vi "Live Display and capture_4.vi"() -> ()   [LabVIEW 2020]
doc: "The Acquire Every Image (Optimized Performance) example shows the basics of using a ring acquisition. There are some camera restrictions to using this mode that are described in more detail in the block diagram of the VI, but it is recommended to use this method for performance-critical applications when possible."
uses:
  <vilib>/vision/driver/IMAQdx.llb/IMAQdx Acquisition Mode.ctl
  Camera Server/Globals/CamServer global.vi
  <vilib>/vision/driver/NI_Vision_Acquisition_Software.lvlib
  <resource>/objmgr/imaqdx.rc
panel:
  out "Name 4":string
  out "Name 3":string
  out "Name 2":string
  out "Name 1":string
  out "Image 4":T1(plugin-control)
  out "Image 3":T1(plugin-control)
  out "Image 2":T1(plugin-control)
  out "error out":errorcluster
  out "Numeric":i32
  out "Image 1":T1(plugin-control)
  in  "Stop":bool
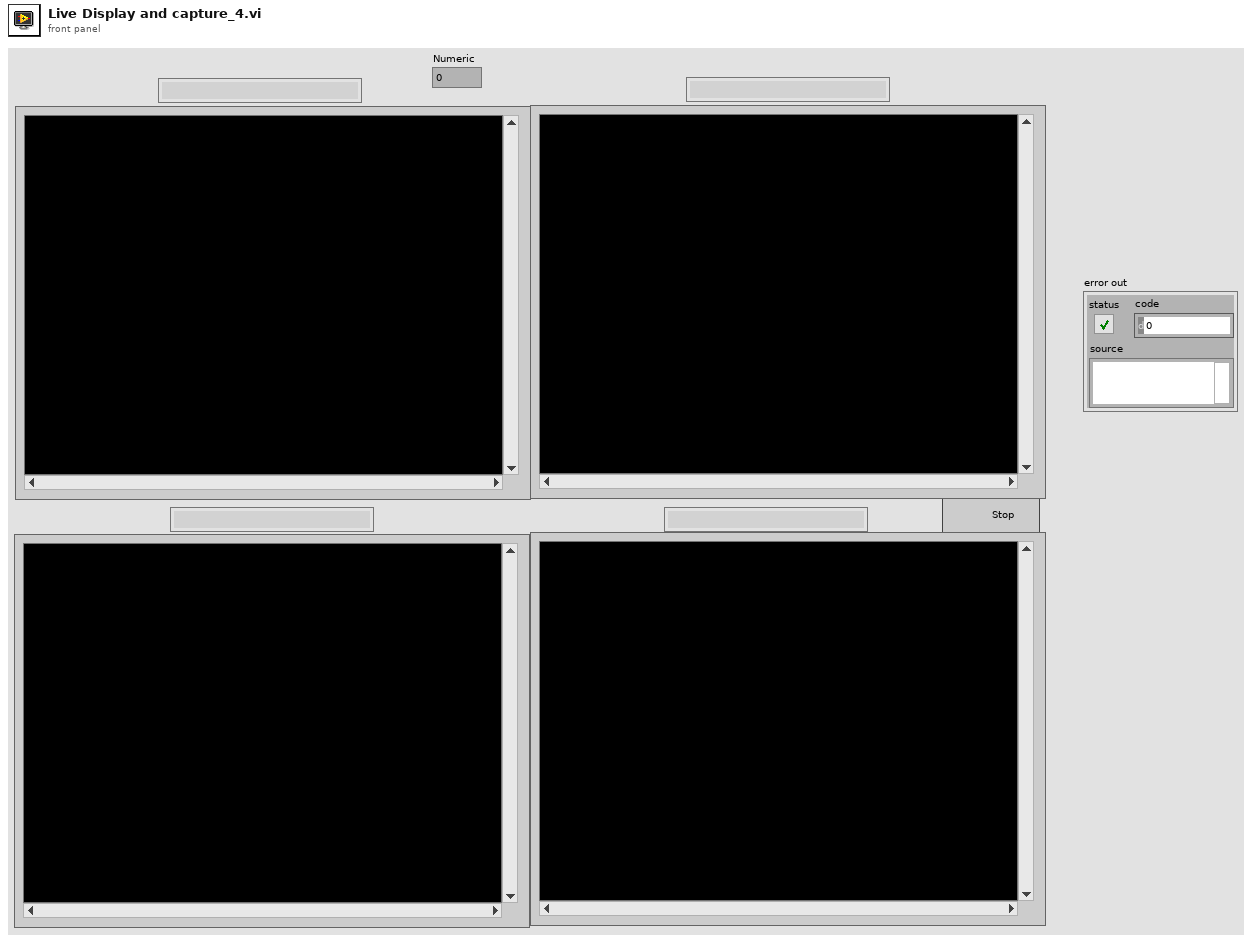
[diagram p1: front panel]
types:
  T1 = typedef "IMAQ Image.ctl" = refnum<image>
  T2 = typedef "NI_Vision_Acquisition_Software.lvlib/IMAQdx Acquisition Mode.ctl" = enum32{"One Shot", "Continuous"}
  T3 = typedef "Camera enum.ctl" = string
  T4 = typedef "IMAQdx.ctl" = refnum<k21>
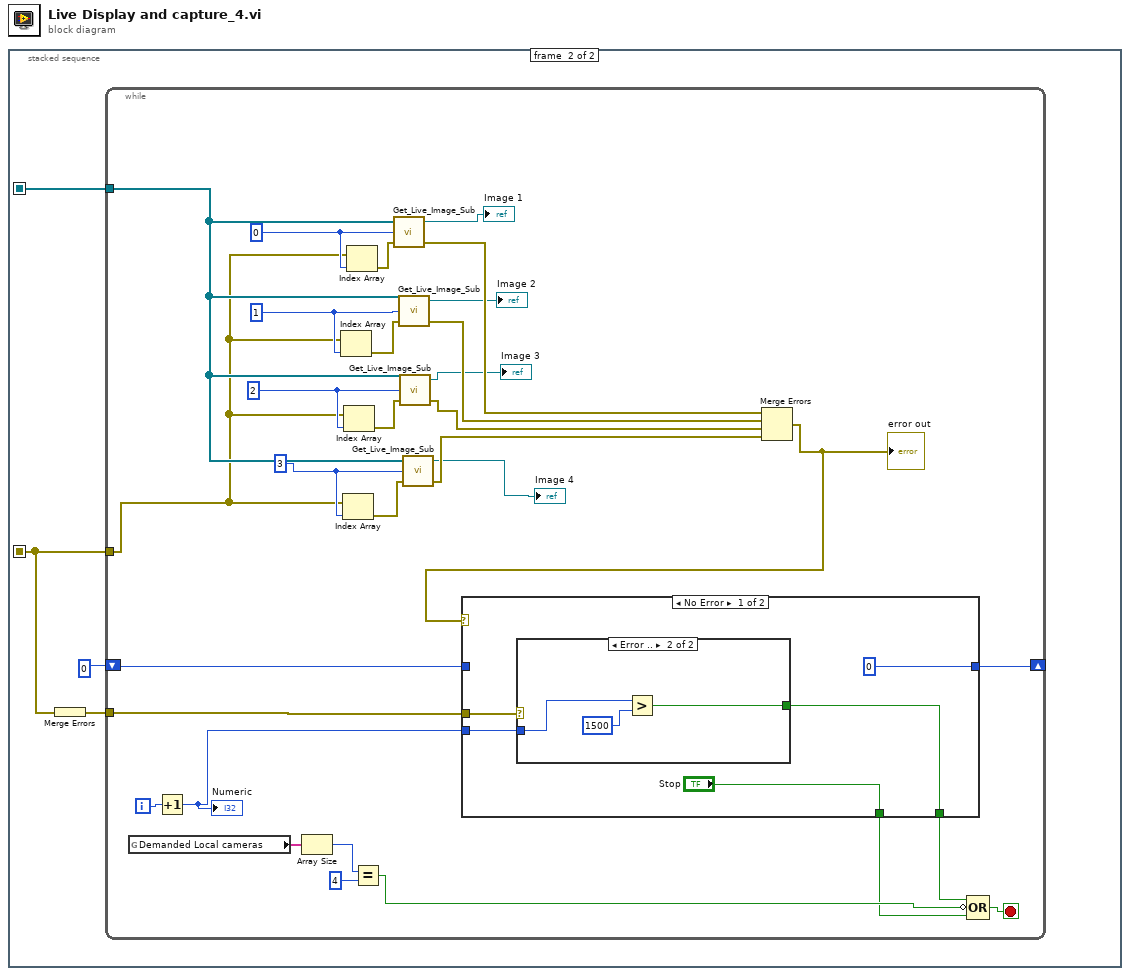
[diagram p0: block diagram]
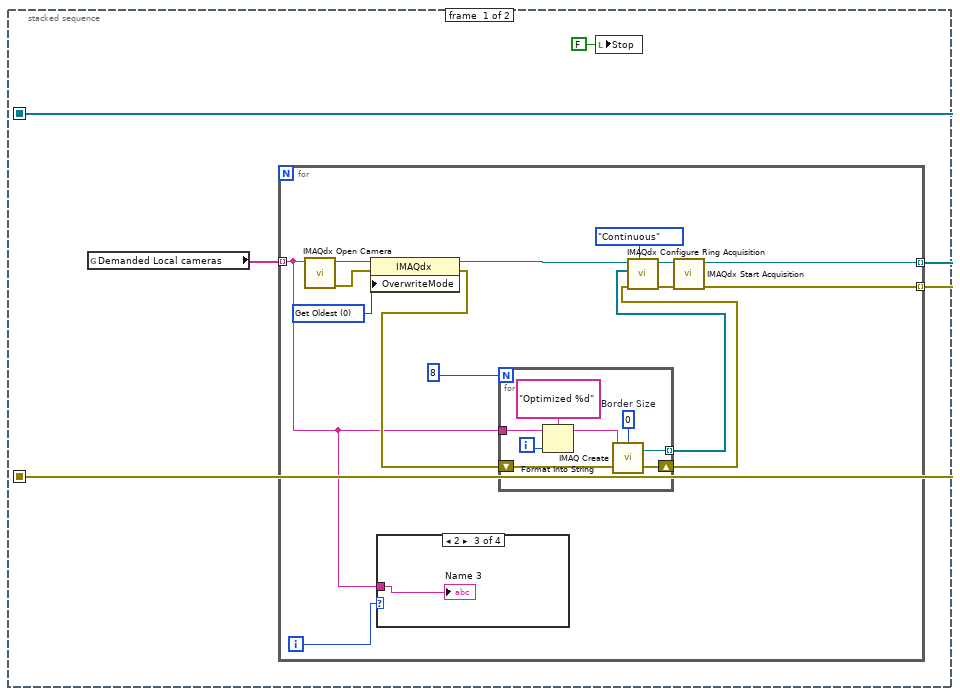
[diagram p2: hidden frame]
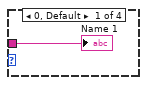
[diagram p3: hidden frame]
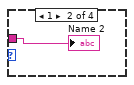
[diagram p4: hidden frame]
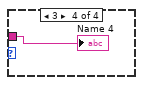
[diagram p5: hidden frame]
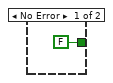
[diagram p6: hidden frame]
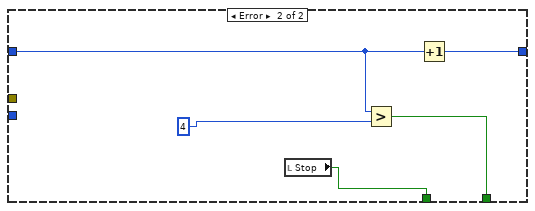
[diagram p7: hidden frame]
diagram:
  n1 = stacked-sequence {
    seq-local: [w4 _] -> [_ w35]
    seq-local: [w3 _] -> [_ w33]
    frame #0 {
      n2 = global read "CamServer global.vi" "Demanded Local cameras"() -> (w2:T3[])
      n3 = for {
        tunnel: w2 -> [w5] mode=indexing
        tunnel: [w13] -> w4 mode=indexing
        tunnel: [w12] -> w3 mode=indexing
        i -> [w6]
        w7 = u32 0 items=["Get Oldest"=0, "Fail"=2, "Get Newest"=3] ("OverwriteMode")
        n4 = call <vilib>:"IMAQdx Open Camera.vi"("Session In"=w5) -> ("error out"=w19:errorcluster, "Session Out"=w18:T4)  [unwired: 2 in, 7 out]
        n5 = property class="IMAQdx"(reference=w18, error in=w19, "OverwriteMode"=w7) -> (reference out=w14:T4, error out=w11:errorcluster)
        n6 = case shown="2" w6 {
          tunnel: w5 -> [w20 w21 w22 w23]
          frame 0, Default {
            "Name 1" <- w20
          }
          frame 1 {
            "Name 2" <- w21
          }
          frame 2 {
            "Name 3" <- w22
          }
          frame 3 {
            "Name 4" <- w23
          }
        }
        n7 = for {
          N: 8 ("Number of Images") -> [_]
          tunnel: [w30] -> w9 mode=indexing
          shift-right: [w29] -> w10
          shift-left: w11 -> [w31]
          tunnel: w5 -> [w24]
          i -> [w28]
          w25 = 0  # Border Size
          n8 = Format Into String(format string="Optimized %d" ("Image Name"), initial string=w24, w28) -> (resulting string=w27:string)  [unwired: 1 in, 1 out]
          n9 = call "IMAQ Create"("Border Size"=w25, "Image Name"=w27, "error in (no error)"=w31) -> ("New Image"=w30:T1, "error out"=w29:errorcluster)  [unwired: 1 in, 1 out]
        }
        n10 = call <vilib>:"IMAQdx Configure Ring Acquisition.vi"("Mode"=IMAQdx_Acquisition_Mode."Continuous" ("Continuous?"), "error in"=w10, "Images"=w9, "Session In"=w14) -> ("error out"=w16:errorcluster, "Session Out"=w15:T4)  [unwired: 5 in, 1 out]
        n11 = call <vilib>:"IMAQdx Start Acquisition.vi"("error in"=w16, "Session In"=w15) -> ("error out"=w12:errorcluster, "Session Out"=w13:T4)  [unwired: 8 out]
      }
      n12 = local write "Stop"(FALSE ("Stop")) -> ()
    }
    frame #1 {
      n13 = Merge Errors(w33) -> (w32:errorcluster)
      n14 = while {
        tunnel: w35 -> [w60]
        tunnel: w33 -> [w41]
        shift-right: [w51] -> _
        shift-left: 0 -> [w50]
        tunnel: w32 -> [w39]
        i -> [w65]
        stop <- w66 stop-if-true
        w49 = 3 ("y")
        w45 = 2 ("y")
        w46 = 1 ("y")
        w47 = 0 ("y")
        n15 = global read "CamServer global.vi" "Demanded Local cameras"() -> (w64:T3[])
        n16 = Increment(x=w65) -> (x+1=w38:i32)
        "Numeric" <- w38
        n17 = Array Size(array=w64) -> (size(s)=w63:i32)
        n18 = Index Array(array=w41, index=w46) -> (element=w43:errorcluster)
        n19 = Index Array(array=w41, index=w49) -> (element=w48:errorcluster)
        n20 = Index Array(array=w41, index=w45) -> (element=w44:errorcluster)
        n21 = Index Array(array=w41, index=w47) -> (element=w42:errorcluster)
        n22 = Equal?(x=w63, y=4) -> (x = y?=w62:bool)
        n23 = call "Get_Live_Image_Sub.vi"("error in"=w42, "index"=w47, "Session Array"=w60) -> ("error out"=w56:errorcluster, "Image"=→"Image 1":T1)  [unwired: 1 in]
        n24 = call "Get_Live_Image_Sub.vi"("error in"=w43, "index"=w46, "Session Array"=w60) -> ("error out"=w57:errorcluster, "Image"=→"Image 2":T1)  [unwired: 1 in]
        n25 = call "Get_Live_Image_Sub.vi"("error in"=w44, "index"=w45, "Session Array"=w60) -> ("error out"=w58:errorcluster, "Image"=→"Image 3":T1)  [unwired: 1 in]
        n26 = call "Get_Live_Image_Sub.vi"("error in"=w48, "index"=w49, "Session Array"=w60) -> ("error out"=w59:errorcluster, "Image"=→"Image 4":T1)  [unwired: 1 in]
        n27 = Merge Errors(w56, w57, w58, w59) -> (w40:errorcluster)
        "error out" <- w40
        n28 = case shown="No Error" w40 {
          tunnel: [0 w80] -> w51
          tunnel: w50 -> [_ w79]
          tunnel: [w68 w78] -> w36
          tunnel: w39 -> [w70 _]
          tunnel: w38 -> [w69 _]
          tunnel: ["Stop" w76] -> w37
          frame No Error {
            n29 = case shown="Error .." w70 {
              tunnel: w69 -> [_ w74]
              tunnel: [FALSE w73] -> w68
              frame No Error {
              }
              frame Error {
                n30 = Greater?(x=w74, y=1500) -> (0:w73:bool)
              }
            }
          }
          frame Error {
            n31 = local read "Stop"() -> (w76:bool)
            n32 = Greater?(x=w79, y=4) -> (0:w78:bool)
            n33 = Increment(x=w79) -> (x+1=w80:i32)
          }
        }
        n34 = Compound Arithmetic op=OR(w36, invert w62, w37) -> (w66:bool)
      }
    }
  }
